vi "Create Channels.vi"(8 "error in":errorcluster, 10 "9226 in":refnum<class "9226.lvclass">, 11 "Parent Ref in":T1 format="%.0x") -> (0 "error out":errorcluster, 2 "9226 out":refnum<class "9226.lvclass">, 3 "Parent Ref out":T1 format="%.0x")   [LabVIEW 2019, in "Modules.lvlib" / "9226.lvclass"]
uses:
  9226.lvclass
  C:/Users/nitest/Desktop/Git 2019/niveristand-scan-engine-module-libraries/Source/RSI Module/RSI Module.lvclass
  <vilib>/NI VeriStand/Custom Device API/Custom Device Item Ref.ctl
  <vilib>/NI VeriStand/Custom Device API/Custom Device Channel Type.ctl
  <vilib>/NI VeriStand/Custom Device API/Custom Device Channel.ctl
  RSI Module/Class Property Strings.vi
  RSI Module/Channel GUIDs.vi
  <vilib>/NI VeriStand/Custom Device API/Custom Device API.lvlib
  RSI Module/RSI Module.lvclass
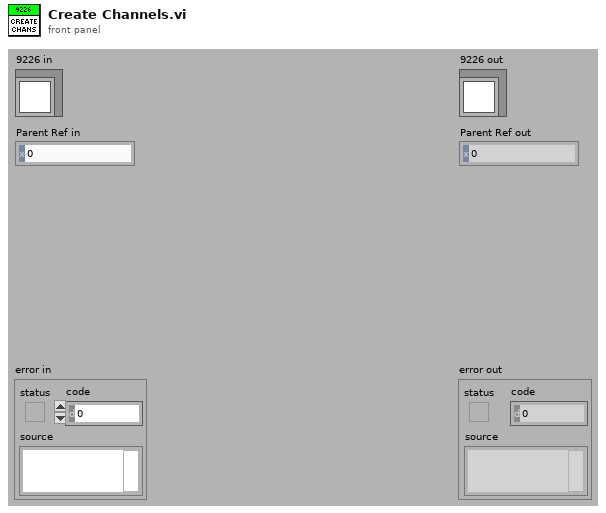
[diagram p1: front panel]
types:
  T1 = typedef "Custom Device API.lvlib/Custom Device Item Ref.ctl" = u64
  T2 = typedef "Custom Device API.lvlib/Custom Device Channel.ctl" = cluster{"Type":T3, "Units":string, "Default Value":dbl, "Faultable":bool, "Scalable":bool}
  T3 = typedef "Custom Device API.lvlib/Custom Device Channel Type.ctl" = enum16{"Input", "Output"}
  T4 = typedef "Modules.lvlib/RSI Module.lvclass/Channels.ctl" = cluster{"# Input Channels":i32, "# Output Channels":i32, "Channel Type":T5, "Units":string}
  T5 = typedef "Modules.lvlib/RSI Module.lvclass/Channel Type.ctl" = enum16{"Analog", "Digital"}
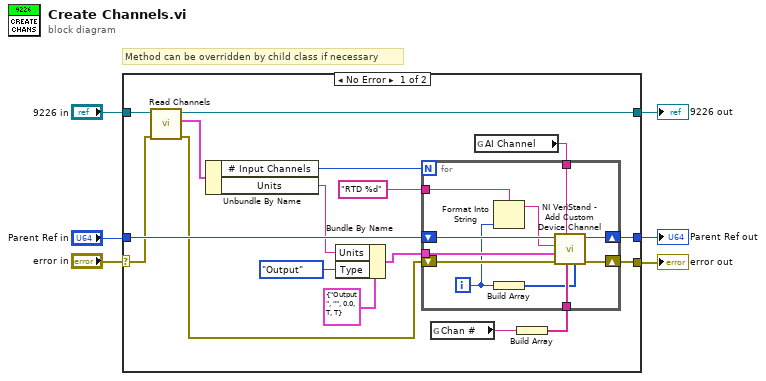
[diagram p0: block diagram]
diagram:
  # "Method can be overridden by child class if necessary"
  n1 = case shown="No Error" "error in" {
    selector: "error in" -> [w16 w37]
    tunnel: [w20 w37] -> w5
    tunnel: [w10 w36] -> w3
    tunnel: "9226 in" -> [w11 w36]
    tunnel: "Parent Ref in" -> [w23 w35]
    tunnel: [w19 w35] -> w1
    frame No Error {
      n2 = call "Read Channels.vi"("error in (no error)"=w16, "RSI Module in"=w11) -> ("error out"=w8:errorcluster, "Channels"=w17:T4, "RSI Module out"=w10:refnum<class "9226.lvclass">)  [unwired: 7 in]
      n3 = Unbundle By Name(w17) -> ("# Input Channels"=w14:i32, "Units"=w18:string)
      n4 = Bundle By Name(cluster=T2 {"Type"=enum."Output", "Units"="", "Default Value"=0.0, "Faultable"=TRUE, "Scalable"=TRUE} ("Channel"), "Units"=w18, "Type"=Custom_Device_Channel_Type."Output") -> (w7:T2)
      n5 = global read "Class Property Strings.vi" "Chan #"() -> (w22:string)
      n6 = global read "Channel GUIDs.vi" "AI Channel"() -> (w13:string)
      n7 = Build Array(w22) -> (w21:string[])
      n8 = for {
        N: w14 -> [_]
        tunnel: w7 -> [w27]
        tunnel: w13 -> [w28]
        tunnel: w21 -> [w32]
        shift-right: [w30] -> w20
        shift-left: w8 -> [w34]
        shift-right: [w29] -> w19
        shift-left: w23 -> [w33]
        tunnel: "RTD %d" ("format string") -> [w26]
        i -> [w25]
        n9 = Format Into String(format string=w26, w25) -> (resulting string=w24:string)  [unwired: 2 in, 1 out]
        n10 = Build Array(w25) -> (w31:i32[])
        n11 = call <vilib>:"NI VeriStand - Add Custom Device Channel.vi"("Property Values"=w31, "Property names"=w32, "GUID (Default Channel)"=w28, "error in (no error)"=w34, "Channel"=w27, "Channel Name"=w24, "Parent Ref in"=w33) -> ("error out"=w30:errorcluster, "Parent Ref out"=w29:T1)  [unwired: 1 in, 2 out]
      }
    }
    frame Error {
    }
  }
  "error out" <- w5
  "9226 out" <- w3
  "Parent Ref out" <- w1
